vi "ParsedData.vi"(8 "error in (no error)":errorcluster, 9 "StdErr":string, 10 "StdOut":string, 11 "Arguments":string) -> (0 "error out":errorcluster, 3 "ParsedData":refnum<class "ParsedData.lvclass">)   [LabVIEW 2022 SP3, in "ArgumentParser.lvlib" / "ParsedData.lvclass"]
uses:
  ParsedData.lvclass
  _Arguments.ctl
  ParsedData.lvclass/ParsedData.ctl
  <vilib>/Utility/error.llb/Trim Whitespace One-Sided.vi
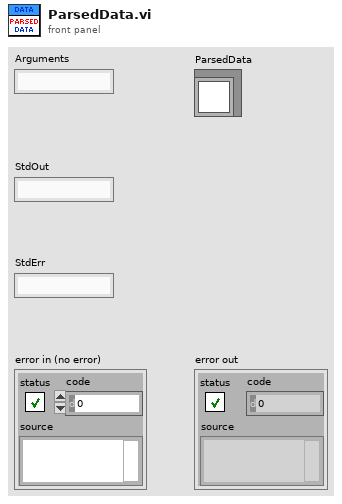
[diagram p1: front panel]
types:
  T1 = typedef "ArgumentParser.lvlib/ParsedData.lvclass/_Arguments.ctl" = map{string, string}
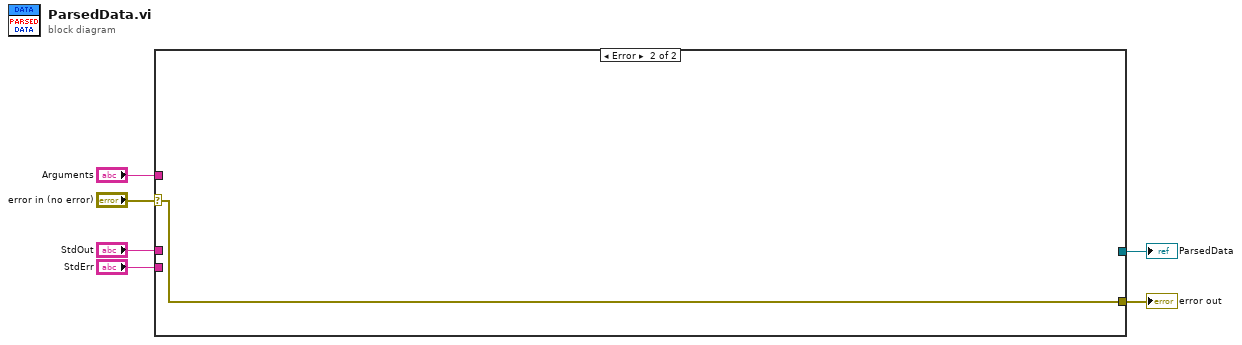
[diagram p0: block diagram]
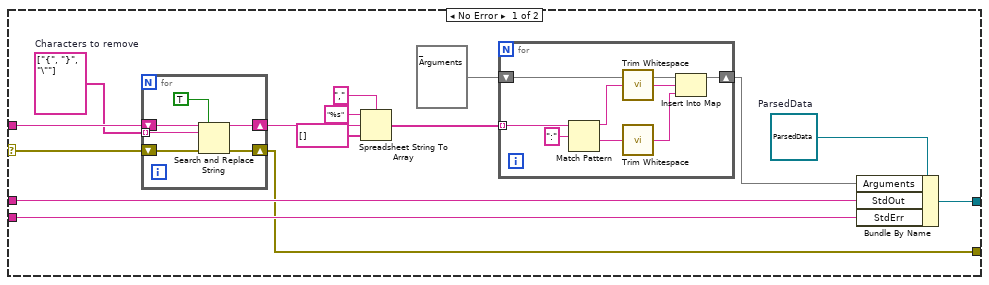
[diagram p2: hidden frame]
diagram:
  n1 = case shown="Error" "error in (no error)" {
    selector: "error in (no error)" -> [w13 w36]
    tunnel: [w12 w36] -> w5
    tunnel: [w20 _] -> w4
    tunnel: "Arguments" -> [w14 _]
    tunnel: "StdOut" -> [w19 _]
    tunnel: "StdErr" -> [w18 _]
    frame No Error {
      w11 = string[] ["{", "}", "\""]  # Characters to remove
      w21 = refnum<class "ParsedData.lvclass"> refnum  # ParsedData
      n2 = for {
        tunnel: w11 -> [w30] mode=indexing
        shift-right: [w35] -> w15
        shift-left: w14 -> [w34]
        shift-right: [w32] -> w12
        shift-left: w13 -> [w33]
        n3 = Search and Replace String(replace all?=TRUE ("replace all? (F)"), input string=w34, search string=w30, error in=w33) -> (result string=w35:string, error out=w32:errorcluster)  [unwired: 4 in, 2 out]
      }
      n4 = Spreadsheet String To Array(delimiter (Tab)=",", format string="%s", spreadsheet string=w15, array type (2D Dbl)=string[] []) -> (array=w10:string[])
      n5 = for {
        tunnel: w10 -> [w25] mode=indexing
        shift-right: [w28] -> w8
        shift-left: T1 {} ("Arguments") -> [w29]
        n6 = Match Pattern(string=w25, regular expression=":" ("search string/char (-)")) -> (before substring=w23:string, after substring=w22:string)  [unwired: 1 in, 2 out]
        n7 = call <vilib>:"Trim Whitespace.vi"("string"=w23) -> ("trimmed string"=w27:string)  [unwired: 1 in]
        n8 = call <vilib>:"Trim Whitespace.vi"("string"=w22) -> ("trimmed string"=w26:string)  [unwired: 1 in]
        n9 = Insert Into Map(map in=w29, key=w27, value=w26) -> (map out=w28:T1)  [unwired: 2 out]
      }
      n10 = Bundle By Name(cluster=w21, "Arguments"=w8, "StdOut"=w19, "StdErr"=w18) -> (w20:refnum<class "ParsedData.lvclass">)
    }
    frame Error {
    }
  }
  "error out" <- w5
  "ParsedData" <- w4
